vi "qDEC.vi"(0 "System no.":i32=1 min=1 max=4 step=1, 2 "Axes to query":string[](array[string]), 3 "All axes?":bool, 4 "Axis identifier?":bool=TRUE, 5 "error in":errorcluster) -> (14 "Deceleration":dbl[](array[numeric]) format="%.6f", 19 "error out":errorcluster)   [LabVIEW 2020]
doc: "Returns closed-loop deceleration setting for specified axes.\n\nC-843, C-867, C-877, C-884, C-891, E-861, E-874, Hydra, Pollux, Mercury_GCS: If All axes? = TRUE, then Axis identifier? can be FALSE. Deceleration unit is mm/s².\n\nE-873: If All axes? = TRUE, then Axis identifier? can be FALSE. Deceleration unit is mm/s²."
panel:
  # "Returns closed-loop deceleration setting for specified axes."
  # "If all axes: use"
  # "Query"
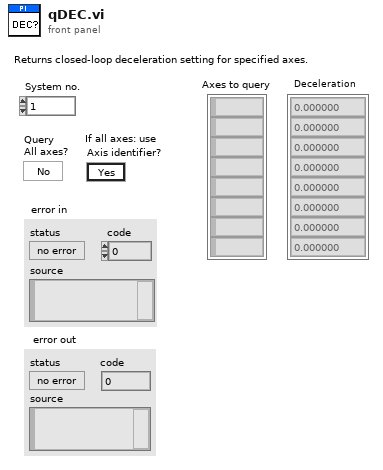
[diagram p1: front panel]
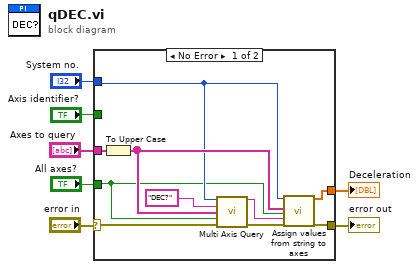
[diagram p0: block diagram]
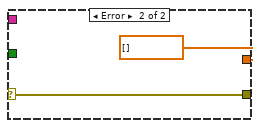
[diagram p2: hidden frame]
diagram:
  n1 = case shown="No Error" "error in" {
    selector: "error in" -> [w11 w18]
    tunnel: [w9 dbl[] [] ("Values")] -> w7
    tunnel: "Axes to query" -> [w13 _]
    tunnel: [w10 w18] -> w5
    tunnel: "Axis identifier?" -> [_ _]
    tunnel: "System no." -> [w12 _]
    tunnel: "All axes?" -> [w8 _]
    frame No Error {
      n2 = To Upper Case(1:w13) -> (0:w15:string[])
      n3 = call "Multi Axis Query.vi"("System no."=w12, "Command"="DEC?", "Axis"=w15, "All axes?"=w8, "error in (no error)"=w11) -> ("Answer"=w14:string, "error out"=w16:errorcluster)  [unwired: 9 in]
      n4 = call "Assign values from string to axes.vi"("System no."=w12, "Queried axes"=w15, "All axes queried?"=w8, "Input String"=w14, "error in"=w16) -> ("Values"=w9:dbl[], "error out"=w10:errorcluster)  [unwired: 4 in, 9 out]
    }
    frame Error {
    }
  }
  "error out" <- w5
  "Deceleration" <- w7
